vi "user32_GetWindowLongA.vi"(8 "error in (no error)":errorcluster, 10 "nIndex":i32, 11 "hWnd":i64) -> (0 "error out":errorcluster, 3 "return":i32)   [LabVIEW 2020]
uses:
  user32.dll
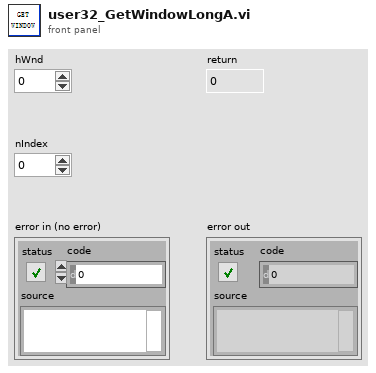
[diagram p1: front panel]
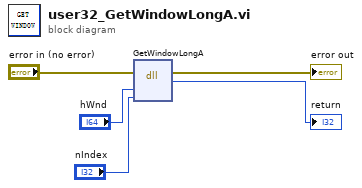
[diagram p0: block diagram]
diagram:
  n1 = dll-call lib="user32.dll" fn="GetWindowLongA"(error in="error in (no error)", "hWnd"="hWnd", "nIndex"="nIndex") -> (error out=→"error out":errorcluster, "返回值"=→"return":i32)  [unwired: 4 in, 1 out]
